vi "Get Child Name[].vi"(8 "error in (no error)":errorcluster, 11 "Doc Class Object[]":refnum<class "Document.lvclass">[](array[class])) -> (0 "error out":errorcluster, 2 "Doc Name[]":string[](array[string]), 3 "Doc Class Object[]":refnum<class "Document.lvclass">[](array[class]))   [LabVIEW 2016, in "Document.lvclass"]
doc: "Get all Child Window Hwnd."
uses:
  Document.lvclass
  Document.lvclass/Document.ctl
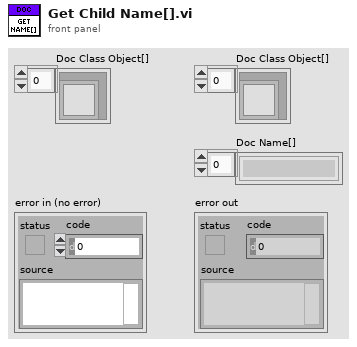
[diagram p1: front panel]
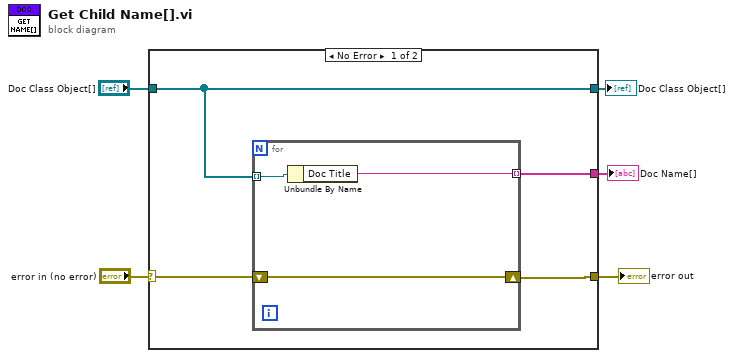
[diagram p0: block diagram]
diagram:
  n1 = case shown="No Error" "error in (no error)" {
    selector: "error in (no error)" -> [w9 w14]
    tunnel: [w8 w14] -> w4
    tunnel: [w7 _] -> w3
    tunnel: "Doc Class Object[]" -> [w6 w13]
    tunnel: [w6 w13] -> w1
    frame No Error {
      n2 = for {
        shift-right: [w12] -> w8
        shift-left: w9 -> [w12]
        tunnel: [w10] -> w7 mode=indexing
        tunnel: w6 -> [w11] mode=indexing
        n3 = Unbundle By Name(w11) -> ("Doc Title"=w10:string)
      }
    }
    frame Error {
    }
  }
  "error out" <- w4
  "Doc Name[]" <- w3
  "Doc Class Object[]" <- w1
